vi "errDetails.vi"() -> ()   [LabVIEW 2020]
uses:
  AIM664LV.lvlib
panel:
  in  "ErrWord":u16
  in  "dimension size":i32
  out "status":i32
  out "ErrStr":string
  out "error out":errorcluster
  in  "error in (no error)":errorcluster
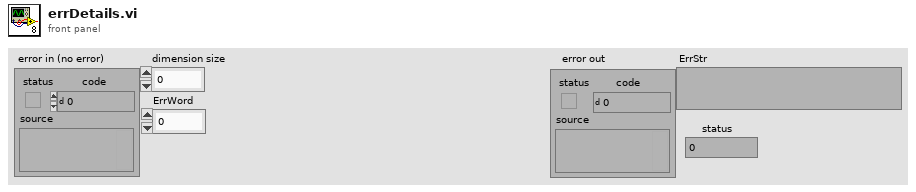
[diagram p1: front panel]
types:
  T1 = cluster{"ErrWord":u16, "ErrStr":string, "ErrStrSize":u8}
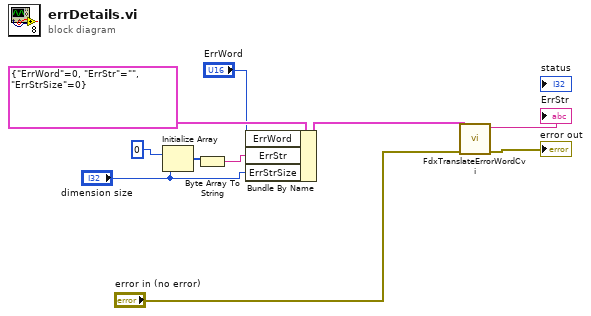
[diagram p0: block diagram]
diagram:
  n1 = Initialize Array(u8 0, "dimension size") -> (w3:u8[])
  n2 = Byte Array To String(unsigned byte array=w3) -> (string=w2:string)
  n3 = Bundle By Name(cluster=T1 {"ErrWord"=0, "ErrStr"="", "ErrStrSize"=0} ("ErrorInfo"), "ErrWord"="ErrWord", "ErrStr"=w2, "ErrStrSize"="dimension size") -> (w6:T1)
  n4 = call "FdxTranslateErrorWordCvi.vi"("error in"="error in (no error)", "ErrorInfo"=w6) -> ("error out"=→"error out":errorcluster, "ErrStr"=→"ErrStr":string)  [unwired: 8 in]
